vi "Destroy.vi"(0 "MLA":refnum<class "MLA.lvclass">, 5 "error in (no error)":errorcluster) -> (14 "MLA":refnum<class "MLA.lvclass">, 19 "error out":errorcluster)   [LabVIEW 2017, in "MLA.lvclass"]
uses:
  MLA.lvclass
  S5Tools/ErrorLog/ErrorLog.lvclass
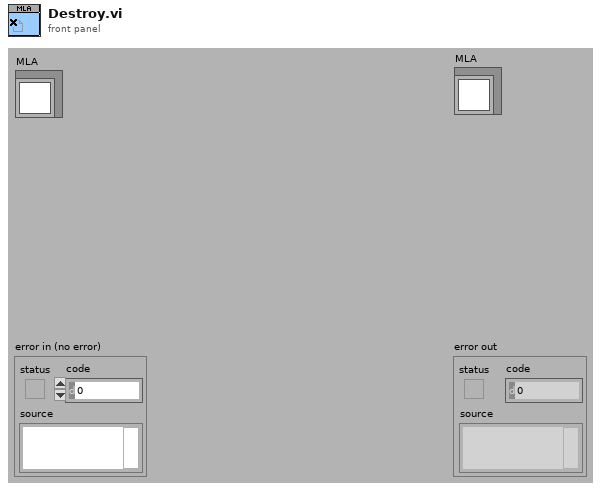
[diagram p1: front panel]
types:
  T1 = typedef "MLA.lvclass/ObjectAttributes.ctl" = cluster{"App Name":string, "App Version":string, "Revision History":string, "Log File Path":path, "Config INI File":path, "Config Path":path, "Log Archive Path":path, "Msg Q's":refnum<queue>[], "VI":refnum<vi>, "ErrLog":refnum<class "ErrorLog.lvclass">}
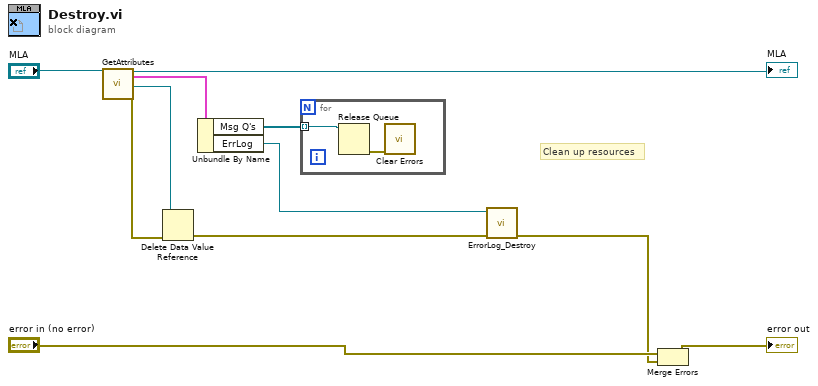
[diagram p0: block diagram]
diagram:
  # "Clean up resources"
  n1 = call "GetAttributes.vi"("MLA"="MLA") -> ("MLA"=→"MLA":refnum<class "MLA.lvclass">, "Data"=w6:T1, "DataRef"=w7:refnum<data-value>, "error out"=w8:errorcluster)  [unwired: 15 in]
  n2 = Delete Data Value Reference(data value reference=w7, error in=w8) -> (error out=w3:errorcluster)  [unwired: 1 out]
  n3 = Unbundle By Name(w6) -> ("Msg Q's"=w4:refnum<queue>[], "ErrLog"=w1:refnum<class "ErrorLog.lvclass">)
  n4 = for {
    tunnel: w4 -> [w13] mode=indexing
    n5 = Release Queue(queue=w13) -> (error out=w12:errorcluster)  [unwired: 2 in, 2 out]
    n6 = call <vilib>:"Clear Errors.vi"("error in (no error)"=w12) -> ()  [unwired: 5 in, 2 out]
  }
  n7 = call-dynamic "ErrorLog_Destroy.vi"("error in (no error)"=w3, "reference in"=w1) -> ("error out"=w2:errorcluster)  [unwired: 8 in, 1 out]
  n8 = Merge Errors("error in (no error)", w2) -> (→"error out":errorcluster)
